vi "Create Upload Segment Response Message.vi"(11 "Service Data Object in":refnum<class "Service Data Object.lvclass">) -> (2 "Response Message":refnum<class "CANopen Response Message.lvclass">, 3 "Service Data Object out":refnum<class "Service Data Object.lvclass">)   [LabVIEW 2024, in "CANopen Master.lvlib" / "Service Data Object.lvclass"]
uses:
  Service Data Object.lvclass
  CANopen Response/CANopen Response Message.lvclass
  Service Data Object.lvclass/Service Data Object.ctl
  CANopen Message/CANopen Message.lvclass
  CANopen/FunctionCode.ctl
  CANopen Master.lvlib
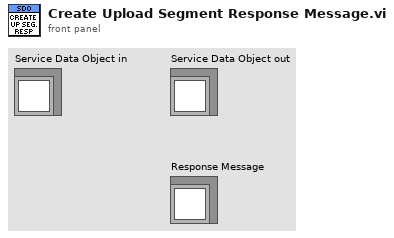
[diagram p1: front panel]
types:
  T1 = typedef "CANopen Master.lvlib/FunctionCode.ctl" = u16
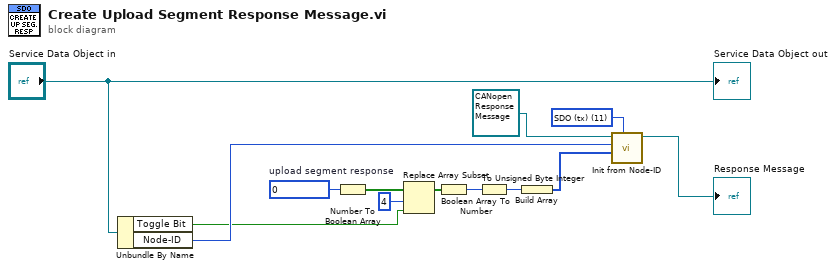
[diagram p0: block diagram]
diagram:
  w5 = u8 0  # upload segment response
  w12 = T1 11 items=["EMCY"=1, "PDO1 (tx)"=3, "PDO1 (rx)"=4, "PDO2 (tx)"=5, "PDO2 (rx)"=6, "PDO3 (tx)"=7, "PDO3 (rx)"=8, "PDO4 (tx)"=9, "PDO4 (rx)"=10, "SDO (tx)"=11, "SDO (rx)"=12, "NMT error control"=14] ("Function code")
  n1 = Unbundle By Name("Service Data Object in") -> ("Toggle Bit"=w4:bool, "Node-ID"=w11:u8)
  n2 = Number To Boolean Array(number=w5) -> (Boolean array=w9:bool[])
  n3 = Replace Array Subset(array=w9, new element=w4, index=4) -> (w7:bool[])
  n4 = Boolean Array To Number(Boolean array=w7) -> (number=w6:u32)
  n5 = To Unsigned Byte Integer(number=w6) -> (unsigned 8bit integer=w2:u8)
  n6 = Build Array(w2) -> (w1:u8[])
  n7 = call "Init from Node-ID.vi"("Function code"=w12, "Data"=w1, "Node-ID"=w11, "CANopen Message in"=refnum<class "CANopen Response Message.lvclass"> refnum ("CANopen Master.lvlib:CANopen Response Message.lvclass")) -> ("CANopen Message out"=→"Response Message":refnum<class "CANopen Response Message.lvclass">)  [unwired: 7 in]
  "Service Data Object out" <- "Service Data Object in"
